vi "Write Timer.vi"(8 "error in (no error)":errorcluster, 10 "Timer":u32, 11 "State Machine in":refnum<class "CCS_State Machine.lvclass">) -> (0 "error out":errorcluster, 3 "State Machine out":refnum<class "CCS_State Machine.lvclass">)   [LabVIEW 2018, in "CCS_State Machine.lvclass"]
uses:
  CCS_State Machine.lvclass
  CCS_State Machine.lvclass/CCS_State Machine.ctl
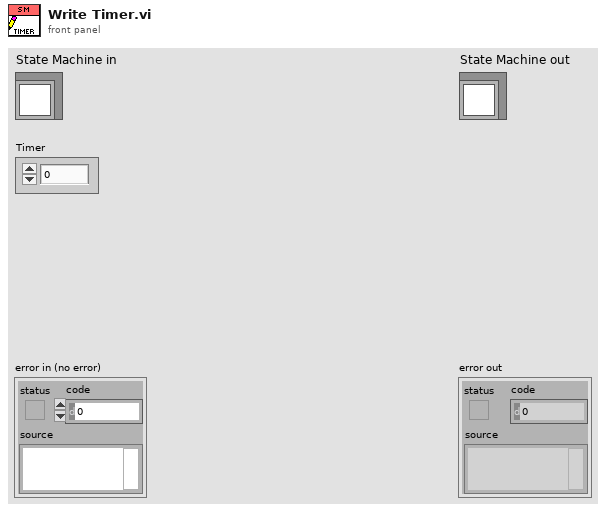
[diagram p1: front panel]
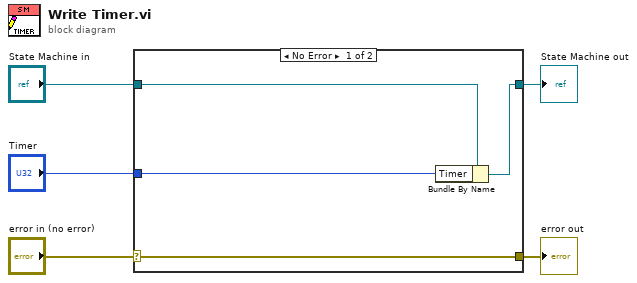
[diagram p0: block diagram]
diagram:
  n1 = case shown="No Error" "error in (no error)" {
    selector: "error in (no error)" -> [w9 w10]
    tunnel: [w9 w10] -> w4
    tunnel: [w7 w11] -> w2
    tunnel: "State Machine in" -> [w8 w11]
    tunnel: "Timer" -> [w6 _]
    frame No Error {
      n2 = Bundle By Name(cluster=w8, "Timer"=w6) -> (w7:refnum<class "CCS_State Machine.lvclass">)
    }
    frame Error {
    }
  }
  "error out" <- w4
  "State Machine out" <- w2
